vi "Beep if saturation.vi"(8 "error in":errorcluster, 9 "Sat Level":sgl, 10 "Beep If Sat.":bool, 11 "Max":sgl) -> (0 "error out":errorcluster)   [LabVIEW 2020]
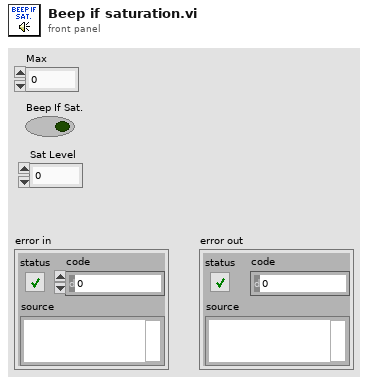
[diagram p1: front panel]
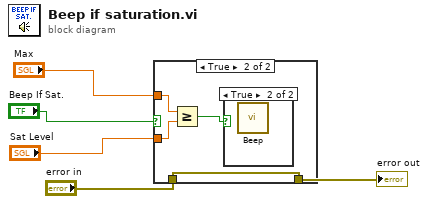
[diagram p0: block diagram]
diagram:
  n1 = case shown="True" "Beep If Sat." {
    tunnel: "Max" -> [_ w10]
    tunnel: "Sat Level" -> [_ w8]
    tunnel: "error in" -> [w6 w7]
    tunnel: [w6 w7] -> w5
    frame False {
    }
    frame True {
      n2 = Greater Or Equal?(x=w10, y=w8) -> (x >= y?=w9:bool)
      n3 = case shown="True" w9 {
        frame False {
        }
        frame True {
          n4 = call <vilib>:"Beep.vi"() -> ()  [unwired: 12 in]
        }
      }
    }
  }
  "error out" <- w5
